vi "Main.vi"(11 "Module Admin":refnum<class "Delacor_lib_QMH_Module Admin.lvclass">) -> ()   [LabVIEW 2019, in "Controller.lvlib"]
doc: "This template is based off of the Queued Message Handler design pattern and the Queued Message Handler project template that ships with LabVIEW.\n\nThe main difference is that the queue is private to this module and communication between modules is performed via Broadcast and Request events.\n\nRequest events are wrapped in public API methods and are handled in the Event Handling Loop (EHL) of this VI. Any module can register for Broadcast events sent by this module. The EHL generates messages based on user interface actions.\n\nThe Message Handling Loop (MHL) processes messages generated by the EHL, or by other messages. The messages are string values, so new messages can be added easily to the Message Cases case structure in the MHL. Each message cluster can also provide an optional value for Message Data, which is a variant that can be converted to whatever message-specific data is required.\n_____\nBased on DQMH Project Template 6.0.0.91."
uses:
  Controller.lvlib
  <vilib>/Delacor/Delacor QMH/Libraries/Module Admin_class/Delacor_lib_QMH_Module Admin.lvclass
  Module Data--cluster.ctl
  <vilib>/Delacor/Delacor QMH/Libraries/Message Queue_class/Delacor_lib_QMH_Message Queue.lvclass/Delacor_lib_QMH_Message Queue.ctl
  Stop Argument--cluster.ctl
  <vilib>/Delacor/Delacor QMH/Libraries/Module Admin_class/Delacor_lib_QMH_Module Admin.lvclass/Delacor_lib_QMH_Module Admin.ctl
  <vilib>/Delacor/Delacor QMH/Libraries/Message Queue_class/Delacor_lib_QMH_Enqueue Message (Single).vi
  <vilib>/Delacor/Delacor QMH/Libraries/Module Admin_class/Delacor_lib_QMH_Get External Launch.vi
  <vilib>/Utility/error.llb/Error Cluster From Error Code.vi
  <vilib>/ErrorRing/Error Ring.xnode
  <vilib>/Delacor/Delacor QMH/Libraries/Message Queue_class/Delacor_lib_QMH_Message Queue.lvclass
  Server/Server.lvlib
panel:
  in  "Connect":bool
  in  "Disconnect":bool
  in  "Subpanel Ref":refnum<vi>
  out "Connected?":bool
  out "error out":errorcluster
  out "Status":string
  in  "Simulate MHL Error":bool
  in  "Simulate EHL Error":bool
  # "Controller"
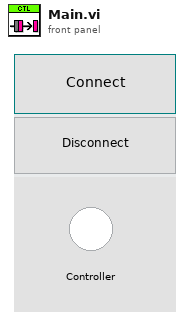
[diagram p1: front panel]
types:
  T1 = typedef "Controller.lvlib/Request Events--cluster.ctl" = cluster{"Stop Module":refnum<user-event>, "Show Panel":refnum<user-event>, "Hide Panel":refnum<user-event>, "Get Module Execution Status":refnum<user-event>, "Show Diagram":refnum<user-event>}
  T2 = typedef "Controller.lvlib/Module Data--cluster.ctl" = cluster{"Status":string}
  T3 = enum32{"invalid lock state", "Not Locked", "Locked (No Password)", "Password-protected"}
  T4 = typedef "Controller.lvlib/Stop Argument--cluster.ctl" = cluster{"Origin":string, "Exit via Stop Module Req?":bool, "Wait for Module to stop?":bool}
  T5 = enum32{"Invalid", "Standard", "Closed", "Hidden", "Minimized", "Maximized"}
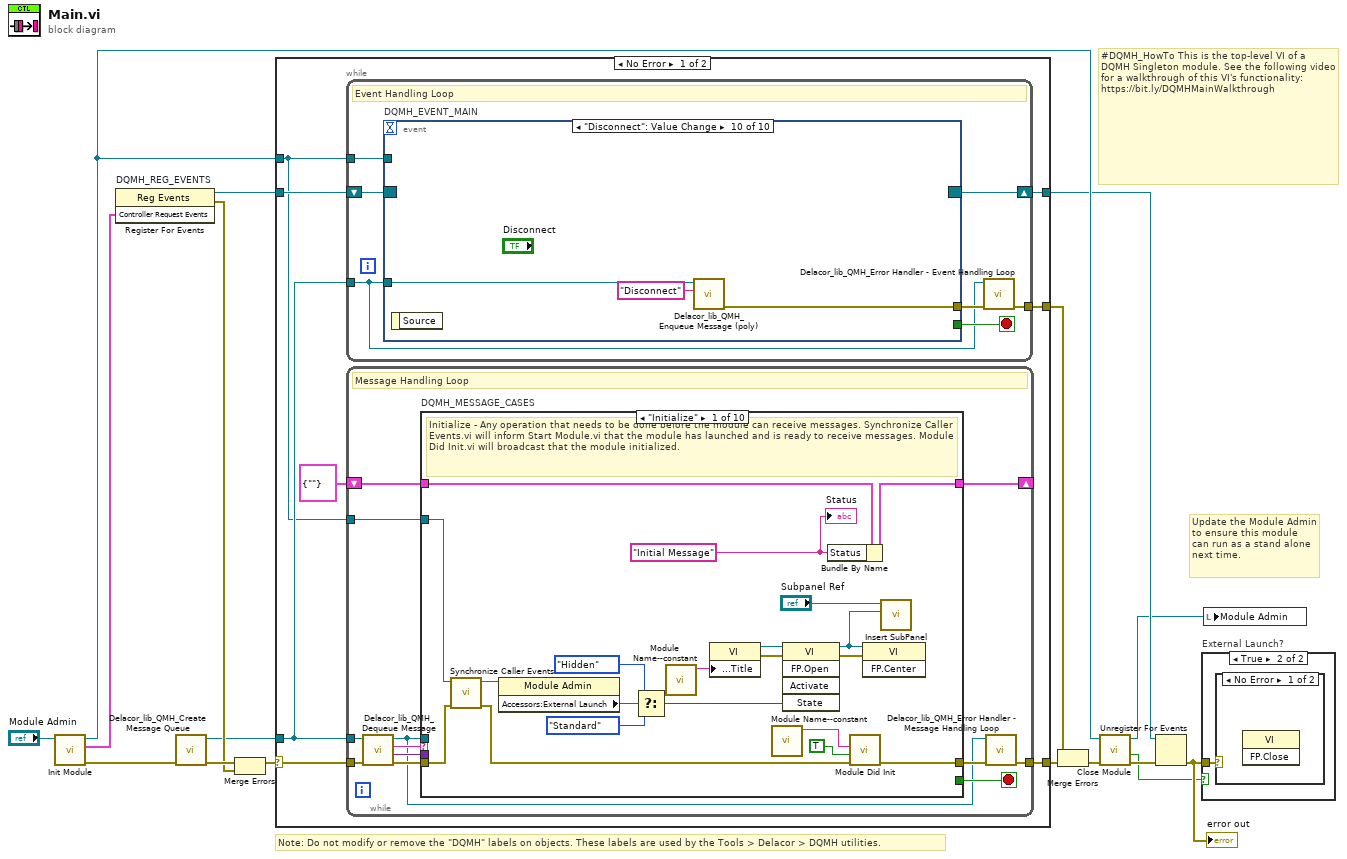
[diagram p0: block diagram]
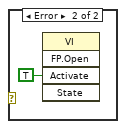
[diagram p3: hidden frame]
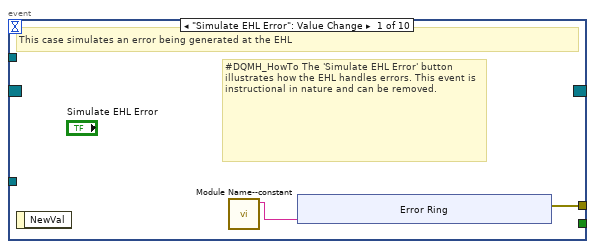
[diagram p4: hidden frame]
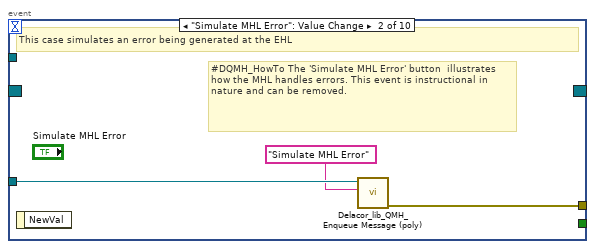
[diagram p5: hidden frame]
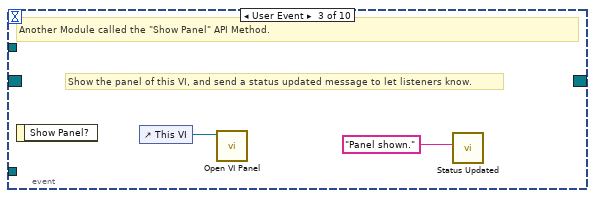
[diagram p6: hidden frame]
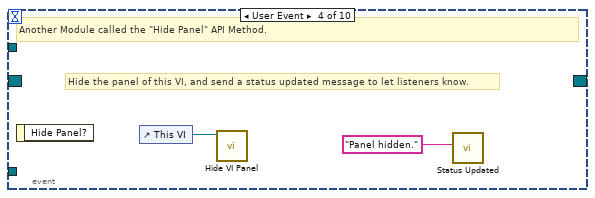
[diagram p7: hidden frame]
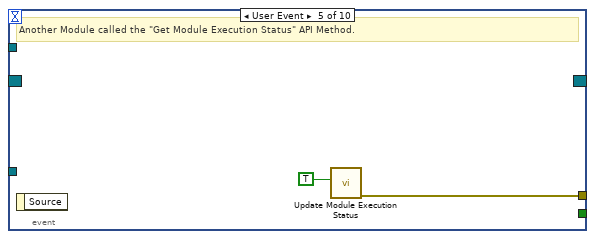
[diagram p8: hidden frame]
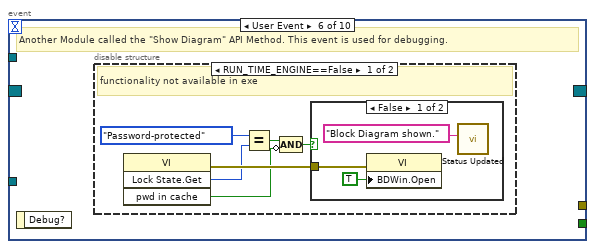
[diagram p9: hidden frame]
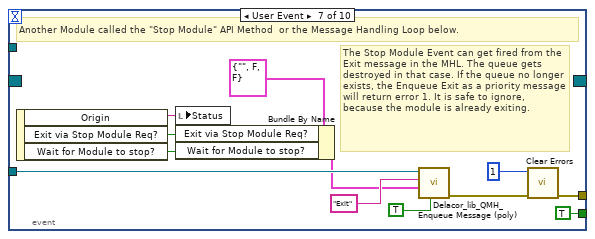
[diagram p12: hidden frame]
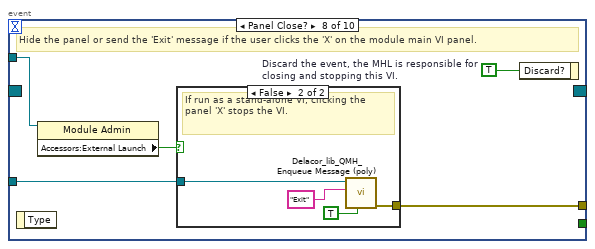
[diagram p13: hidden frame]
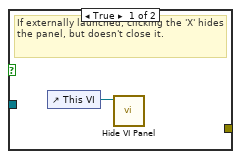
[diagram p14: hidden frame]
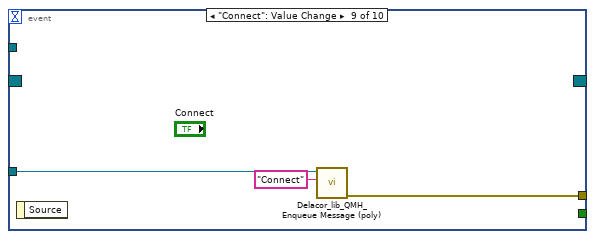
[diagram p15: hidden frame]
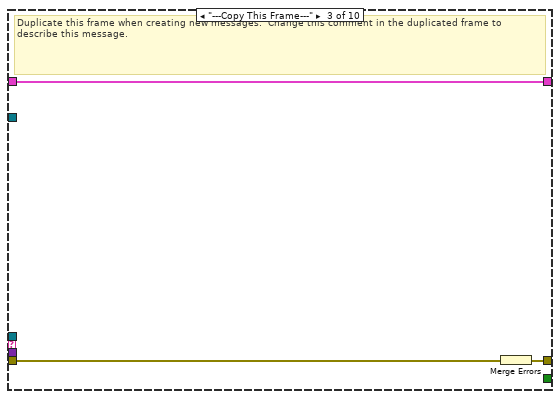
[diagram p17: hidden frame]
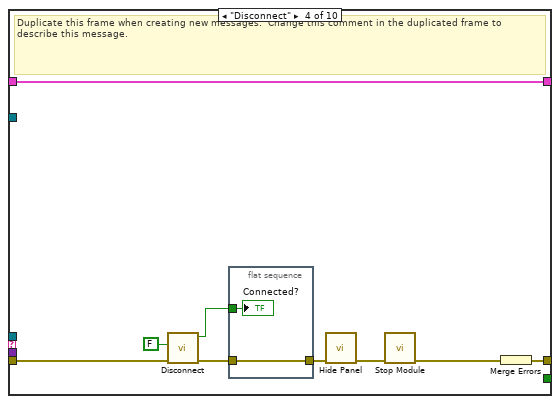
[diagram p18: hidden frame]
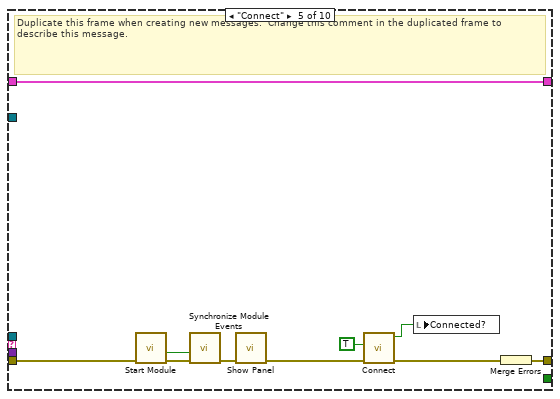
[diagram p19: hidden frame]
diagram:
  # "#DQMH_HowTo This is the top-level VI of a DQMH Singleton module. See the following video for a walkthrough of this VI's functionality: https://bit.ly/DQMHMainWalkthrough"
  # "Note: Do not modify or remove the \"DQMH\" labels on objects. These labels are used by the Tools > Delacor > DQMH utilities."
  # "Update the Module Admin to ensure this module can run as a stand alone next time."
  n1 = call "Init Module.vi"("Singleton Module Admin in"="Module Admin") -> ("error out"=w16:errorcluster, "Controller Request Events"=w5:T1, "Singleton Module Admin out"=w8:refnum<class "Delacor_lib_QMH_Module Admin.lvclass">)  [unwired: 8 in]
  n2 = register-events "DQMH_REG_EVENTS"(w5) -> (reference out=w6:refnum<event-registration>, error out=w9:errorcluster)  [unwired: 2 in]
  n3 = call <vilib>:"Delacor_lib_QMH_Create Message Queue.vi"("error in"=w16) -> ("error out"=w11:errorcluster, "Message Queue"=w4:refnum<class "Delacor_lib_QMH_Message Queue.lvclass">)  [unwired: 9 in]
  n4 = Merge Errors(w11, w9) -> (w10:errorcluster)
  n5 = case shown="No Error" w10 {
    selector: w10 -> [w23 w207]
    tunnel: [w25 w206] -> w17
    tunnel: [w22 w212] -> w7
    tunnel: w6 -> [w20 w212]
    tunnel: w4 -> [w19 w205]
    tunnel: [w24 _] -> w14
    tunnel: w8 -> [w18 w208]
    frame No Error {
      n6 = while {
        tunnel: w19 -> [w26]
        shift-right: [w29] -> w22
        shift-left: w20 -> [w30]
        tunnel: [w31] -> w24
        tunnel: w18 -> [w27]
        stop <- w28 stop-if-true
        # "Event Handling Loop"
        n7 = event "DQMH_EVENT_MAIN" shown="[9] \"Disconnect\": Value Change" {
          selector: w30 -> [_ _ _ _ _ _ _ _ _ _]
          dyn-events: [_ _ _ _ _ _ _ _ _ _] -> w29
          timeout: _ -> [_ _ _ _ _ _ _ _ _ _]
          tunnel: [_ _ _ _ _ _ TRUE ("Discard?") _ _ _] -> w28
          tunnel: w26 -> [_ w43 _ _ _ _ w67 w74 w84 w87]
          tunnel: [w34 w44 _ _ w50 _ w70 w76 w83 w86] -> w32
          tunnel: w27 -> [_ _ _ _ _ _ _ w73 _ _]
          event "Simulate EHL Error": Value Change {
            # "#DQMH_HowTo The 'Simulate EHL Error' button  illustrates how the EHL handles errors. This event is instructional in nature and can be removed."
            # "This case simulates an error being generated at the EHL"
            n8 = event-data() -> ()  [unwired: 1 in, 1 out]
            n9 = call "Module Name--constant.vi"() -> ("Module Name"=w33:string)  [unwired: 11 in]
            n10 = xnode "Error Ring"("parameter 0"=w33) -> ("error out"=w34:errorcluster)
          }
          event "Simulate MHL Error": Value Change {
            # "#DQMH_HowTo The 'Simulate MHL Error' button  illustrates how the MHL handles errors. This event is instructional in nature and can be removed."
            # "This case simulates an error being generated at the EHL"
            n11 = event-data() -> ()  [unwired: 1 in, 1 out]
            n12 = call-poly <vilib>:"Delacor_lib_QMH_Enqueue Message (poly).vi"("Message"="Simulate MHL Error", "Message Queue in"=w43) -> ("error out"=w44:errorcluster)  [unwired: 8 in, 1 out]
          }
          event User Event {
            # "Show the panel of this VI, and send a status updated message to let listeners know."
            # "Another Module called the \"Show Panel\" API Method."
            n13 = event-data() -> ()  [unwired: 1 in, 1 out]
            n14 = control-ref of="This VI"() -> (w46:refnum<vi>)
            n15 = call "Open VI Panel.vi"("VI"=w46) -> ()  [unwired: 10 in, 1 out]
            n16 = call "Status Updated.vi"("Status"="Panel shown." ("format string")) -> ()  [unwired: 10 in, 1 out]
          }
          event User Event {
            # "Hide the panel of this VI, and send a status updated message to let listeners know."
            # "Another Module called the \"Hide Panel\" API Method."
            n17 = event-data() -> ()  [unwired: 1 in, 1 out]
            n18 = control-ref of="This VI"() -> (w48:refnum<vi>)
            n19 = call "Hide VI Panel.vi"("VI"=w48) -> ()  [unwired: 10 in, 1 out]
            n20 = call "Status Updated.vi"("Status"="Panel hidden." ("format string")) -> ()  [unwired: 10 in, 1 out]
          }
          event User Event {
            # "Another Module called the \"Get Module Execution Status\" API Method."
            n21 = event-data() -> ()  [unwired: 1 in, 1 out]
            n22 = call "Update Module Execution Status.vi"("Running?"=TRUE) -> ("error out"=w50:errorcluster)  [unwired: 10 in]
          }
          event User Event {
            # "Another Module called the \"Show Diagram\" API Method. This event is used for debugging."
            n23 = event-data() -> ()  [unwired: 1 in, 1 out]
            n24 = disable-structure shown="RUN_TIME_ENGINE==False" {
              frame condition #0 (active) {
                # "functionality not available in exe"
                n25 = invoke class="VI" method="Lock State.Get"() -> (error out=w56:errorcluster, "Get Lock State"=w55:T3, "pwd in cache"=w52:bool)  [unwired: 4 in, 1 out]
                n26 = Equal?(x=T3."Password-protected", y=w55) -> (x = y?=w53:bool)
                n27 = Compound Arithmetic op=AND(w53, invert w52) -> (w51:bool)
                n28 = case shown="False" w51 {
                  tunnel: w56 -> [w59 _]
                  frame False {
                    n29 = property class="VI"(error in=w59, "BDWin.Open"=TRUE ("Block Diagram Window:Open")) -> ()  [unwired: 1 in, 2 out]
                    n30 = call "Status Updated.vi"("Status"="Block Diagram shown." ("format string")) -> ()  [unwired: 10 in, 1 out]
                  }
                  frame True {
                    # "Password-protected VI, and the password is not in the cache. Do not show the diagram."
                  }
                }
              }
              frame condition #1 {
              }
            }
          }
          event User Event {
            # "The Stop Module Event can get fired from the Exit message in the MHL. The queue gets destroyed in that case. If the queue no longer exists, the Enqueue Exit as a priority message will return error 1. It is safe to ignore, because the module is already exiting."
            # "Another Module called the \"Stop Module\" API Method  or the Message Handling Loop below."
            n31 = event-data() -> ("Origin"=w66:string, "Exit via Stop Module Req?"=w62:bool, "Wait for Module to stop?"=w61:bool)  [unwired: 1 in]
            n32 = local write "Status"(w66) -> ()
            n33 = Bundle By Name(cluster=T4 {"Origin"="", "Exit via Stop Module Req?"=FALSE, "Wait for Module to stop?"=FALSE} ("Stop Argument"), "Exit via Stop Module Req?"=w62, "Wait for Module to stop?"=w61) -> (w60:T4)
            n34 = call-poly <vilib>:"Delacor_lib_QMH_Enqueue Message (poly).vi"("Priority Message? (F)"=TRUE, "Message Data"=w60, "Message"="Exit", "Message Queue in"=w67) -> ("error out"=w71:errorcluster)  [unwired: 6 in, 1 out]
            n35 = call <vilib>:"Clear Errors.vi"("error in (no error)"=w71, "specific error code to clear (0: all)"=1) -> ("error out"=w70:errorcluster)  [unwired: 4 in, 1 out]
          }
          event Panel Close? {
            w75 = TRUE  # Discard the event, the MHL is responsible for closing and stopping this VI.
            # "Hide the panel or send the 'Exit' message if the user clicks the 'X' on the module main VI panel."
            n36 = event-data() -> ()  [unwired: 1 in, 1 out]
            n37 = property class="Module Admin"(reference=w73) -> ("Accessors:External Launch"=w72:bool)  [unwired: 1 in, 2 out]
            n38 = case shown="False" w72 {
              tunnel: w74 -> [_ w80]
              tunnel: [_ w81] -> w76
              frame True {
                # "If externally launched, clicking the 'X' hides the panel, but doesn't close it."
                n39 = control-ref of="This VI"() -> (w77:refnum<vi>)
                n40 = call "Hide VI Panel.vi"("VI"=w77) -> ()  [unwired: 10 in, 1 out]
              }
              frame False {
                # "If run as a stand-alone VI, clicking the panel 'X' stops the VI."
                n41 = call-poly <vilib>:"Delacor_lib_QMH_Enqueue Message (poly).vi"("Priority Message? (F)"=TRUE, "Message"="Exit", "Message Queue in"=w80) -> ("error out"=w81:errorcluster)  [unwired: 7 in, 1 out]
              }
            }
            n42 = event-data("Discard?"=w75) -> ()  [unwired: 1 in, 1 out]
          }
          event "Connect": Value Change {
            n43 = event-data() -> ()  [unwired: 1 in, 1 out]
            n44 = call-poly <vilib>:"Delacor_lib_QMH_Enqueue Message (poly).vi"("Message"="Connect", "Message Queue in"=w84) -> ("error out"=w83:errorcluster)  [unwired: 8 in, 1 out]
          }
          event "Disconnect": Value Change {
            n45 = event-data() -> ()  [unwired: 1 in, 1 out]
            n46 = call-poly <vilib>:"Delacor_lib_QMH_Enqueue Message (poly).vi"("Message"="Disconnect", "Message Queue in"=w87) -> ("error out"=w86:errorcluster)  [unwired: 8 in, 1 out]
          }
        }
        n47 = call-dynamic "Delacor_lib_QMH_Error Handler - Event Handling Loop.vi"("error in"=w32, "Message Queue in"=w26) -> ("dup error in"=w31:errorcluster)  [unwired: 8 in, 1 out]
      }
      n48 = while {
        tunnel: w19 -> [w90]
        shift-right: [w94] -> _
        shift-left: T2 {"Status"=""} ("Data Cluster") -> [w95]
        tunnel: w23 -> [w98]
        tunnel: [w96] -> w25
        tunnel: w18 -> [w88]
        stop <- w93 stop-if-true
        # "Message Handling Loop"
        n49 = call-dynamic "Delacor_lib_QMH_Dequeue Message.vi"("error in"=w98, "Message Queue in"=w90) -> ("error out"=w97:errorcluster, "Message Data"=w91:variant, "Message"=w92:string, "Message Queue out"=w89:refnum<class "Delacor_lib_QMH_Message Queue.lvclass">)  [unwired: 6 in]
        n50 = case "DQMH_MESSAGE_CASES" shown="\"Initialize\"" w92 {
          selector: w92 -> [_ _ _ _ _ _ _ _ _ w192]
          tunnel: w89 -> [_ _ _ _ _ _ _ w162 w184 _]
          tunnel: w97 -> [w117 w121 w124 w131 w139 w147 w152 w169 w190 w194]
          tunnel: [w115 w121 w123 w133 w145 w147 w151 w165 w187 w195] -> w99
          tunnel: w95 -> [w107 w120 w122 w132 w144 w146 w149 w164 w183 w193]
          tunnel: [w106 w120 w122 w132 w144 w146 w149 w164 w183 w193] -> w94
          tunnel: [_ _ _ _ _ _ _ _ w182 _] -> w93
          tunnel: w91 -> [_ _ _ _ _ _ _ w163 w181 _]
          tunnel: w88 -> [w108 _ _ _ _ _ _ w161 w176 _]
          frame "Initialize" {
            w102 = "Initial Message" ("Initial Message")
            # "Initialize - Any operation that needs to be done before the module can receive messages. Synchronize Caller Events.vi will inform Start Module.vi that the module has launched and is ready to receive messages. Module Did Init.vi will broadcast that the module initialized."
            n51 = call "Synchronize Caller Events.vi"("error in (no error)"=w117, "Singleton Module Admin in"=w108) -> ("error out"=w116:errorcluster, "Singleton Module Admin out"=w103:refnum<class "Delacor_lib_QMH_Module Admin.lvclass">)  [unwired: 8 in]
            n52 = property class="Module Admin"(reference=w103) -> ("Accessors:External Launch"=w112:bool)  [unwired: 1 in, 2 out]
            n53 = Select(t=T5."Hidden" ("State"), s=w112, f=T5."Standard" ("State")) -> (s? t:f=w109:T5)
            n54 = call "Module Name--constant.vi"() -> ("Module Name"=w114:string)  [unwired: 11 in]
            n55 = property class="VI"("Front Panel.Title"=w114) -> (reference out=w113:refnum<vi>, error out=w119:errorcluster)  [unwired: 2 in]
            n56 = call "Module Name--constant.vi"() -> ("Module Name"=w104:string)  [unwired: 11 in]
            n57 = invoke class="VI" method="FP.Open"(reference=w113, error in=w119, "State"=w109) -> (reference out=w101:refnum<vi>, error out=w118:errorcluster)  [unwired: 2 in, 3 out]
            n58 = Bundle By Name(cluster=w107, "Status"=w102) -> (w106:T2)
            n59 = call "Module Did Init.vi"("error in (no error)"=w116, "Initialized?"=TRUE, "Origin"=w104) -> ("error out"=w115:errorcluster)  [unwired: 8 in]
            n60 = invoke class="VI" method="FP.Center"(reference=w101, error in=w118) -> ()  [unwired: 1 in, 3 out]
            n61 = call "Insert SubPanel.vi"("VI Ref"=w101, "Subpanel Ref"="Subpanel Ref") -> ()  [unwired: 9 in, 1 out]
            "Status" <- w102
          }
          frame "---Module Specific---" {
            # "Separator -- The following cases handle messages specific to this Module."
          }
          frame "---Copy This Frame---" {
            # "Duplicate this frame when creating new messages.  Change this comment in the duplicated frame to describe this message."
            n62 = Merge Errors(w124) -> (w123:errorcluster)
          }
          frame "Disconnect" {
            # "Duplicate this frame when creating new messages.  Change this comment in the duplicated frame to describe this message."
            n63 = call "Disconnect.vi"("error in"=w131, "Disconnect"=FALSE) -> ("error out"=w126:errorcluster, "Connected?"=w129:bool)  [unwired: 7 in, 1 out]
            n64 = flat-sequence {
              tunnel: w129 -> [w135]
              tunnel: w126 -> [w134]
              tunnel: [w134] -> w125
              frame #0 {
                "Connected?" <- w135
              }
            }
            n65 = call "Hide Panel.vi"("error in (no error)"=w125) -> ("error out"=w128:errorcluster)  [unwired: 10 in]
            n66 = call "Stop Module.vi"("error in"=w128) -> ("error out"=w127:errorcluster)  [unwired: 10 in]
            n67 = Merge Errors(w127) -> (w133:errorcluster)
          }
          frame "Connect" {
            # "Duplicate this frame when creating new messages.  Change this comment in the duplicated frame to describe this message."
            n68 = call "Start Module.vi"("error in (no error)"=w139) -> ("error out"=w140:errorcluster, "Wait for Event Sync?"=w138:bool)  [unwired: 7 in, 2 out]
            n69 = call "Synchronize Module Events.vi"("error in"=w140, "Wait for Event Sync?"=w138) -> ("error out"=w137:errorcluster)  [unwired: 9 in]
            n70 = call "Show Panel.vi"("error in (no error)"=w137) -> ("error out"=w136:errorcluster)  [unwired: 10 in]
            n71 = call "Connect.vi"("error in"=w136, "Connect"=TRUE) -> ("error out"=w142:errorcluster, "Connected?"=w141:bool)  [unwired: 7 in, 1 out]
            n72 = local write "Connected?"(w141) -> ()
            n73 = Merge Errors(w142) -> (w145:errorcluster)
          }
          frame "---Exit and Error Handling---" {
            # "Separator - The following cases handle errors and exit messages."
          }
          frame "Simulate MHL Error" {
            # "#DQMH_HowTo The 'Simulate MHL Error' button  illustrates how the MHL handles errors. This event is instructional in nature and can be removed."
            # "Simulate an error occurring at the MHL"
            n74 = call "Module Name--constant.vi"() -> ("Module Name"=w148:string)  [unwired: 11 in]
            n75 = xnode "Error Ring"("parameter 0"=w148) -> ("error out"=w150:errorcluster)
            n76 = Merge Errors(w152, w150) -> (w151:errorcluster)
          }
          frame "Error" {
            # "#CodeRecommended - If you ever change the name of this \"Error\" message, you'll need to update the name in the Check Loop Error.vi as well."
            # "#CodeRecommended - If the module is running in standalone mode (External Launch = FALSE), this code will pop up an error dialog and call the 'Exit' message if an error occurs. Add more fine-grained error handling here."
            # "Error - Check the error message data and respond accordingly. This message is sent by the \"Error Handler\" VIs at the end of each loop in this application."
            n77 = property class="Module Admin"(reference=w161) -> ("Accessors:External Launch"=w160:bool)  [unwired: 1 in, 2 out]
            n78 = Variant To Data(error in=w169, type=errorcluster {"status"=FALSE, "code"=0, "source"=""} ("error constant"), Variant=w163) -> (data=w170:errorcluster, error out=w167:errorcluster)
            n79 = call "Error Reported.vi"("Error"=w170) -> ()  [unwired: 10 in, 1 out]
            n80 = case shown="False" w160 {
              tunnel: [w175 _] -> w166
              tunnel: w162 -> [w173 _]
              tunnel: w170 -> [w174 _]
              frame False {
                # "If the module is running standalone, then pop up an error dialog and call the \"Exit\" message."
                n81 = call <vilib>:"Simple Error Handler.vi"("error in (no error)"=w174) -> ()  [unwired: 4 in, 5 out]
                n82 = call-poly <vilib>:"Delacor_lib_QMH_Enqueue Message (poly).vi"("Priority Message? (F)"=TRUE, "Message"="Exit", "Message Queue in"=w173) -> ("error out"=w175:errorcluster)  [unwired: 7 in, 1 out]
              }
              frame True {
                # "If the module was launched externally, calling the Error Reported broadcast VI is the only action performed by the \"Error\" message. The module's caller can then process the error appropriately."
              }
            }
            n83 = Merge Errors(w167, w166) -> (w165:errorcluster)
            n84 = local write "error out"(w165) -> ()
          }
          frame "Exit" {
            w180 = 91  # 91: not all Exit messages will have an argument
            w182 = TRUE  # Stop the VI
            # "Release the message queue reference"
            # "#CodeNeeded - Add any required cleanup code here"
            # "Exit - Exit the application."
            n85 = Variant To Data(error in=w190, type=T4 {"Origin"="", "Exit via Stop Module Req?"=FALSE, "Wait for Module to stop?"=FALSE} ("Stop Argument"), Variant=w181) -> (data=w178:T4, error out=w186:errorcluster)
            n86 = call <vilib>:"Clear Errors.vi"("error in (no error)"=w186, "specific error code to clear (0: all)"=w180) -> ("error out"=w189:errorcluster)  [unwired: 4 in, 1 out]
            n87 = control-ref of="This VI"() -> (w177:refnum<vi>)
            n88 = call-dynamic "Delacor_lib_QMH_Release Message Queue.vi"("error in"=w189, "Message Queue"=w184) -> ("error out"=w188:errorcluster)  [unwired: 9 in]
            n89 = call "Handle Exit.vi"("Stop Argument"=w178, "Admin in"=w176, "VI reference"=w177) -> ("error out"=w185:errorcluster)  [unwired: 7 in, 1 out]
            n90 = Merge Errors(w188, w185) -> (w187:errorcluster)
          }
          frame Default {
            # "'Default' case only runs if there is a message that isn't defined in any of the other cases.  Output a programming error."
            n91 = call "Module Name--constant.vi"() -> ("Module Name"=w191:string)  [unwired: 11 in]
            n92 = xnode "Error Ring"("parameter 0"=w192, "parameter 1"=w191) -> ("error out"=w196:errorcluster)
            n93 = Merge Errors(w194, w196) -> (w195:errorcluster)
          }
        }
        n94 = call-dynamic "Delacor_lib_QMH_Error Handler - Message Handling Loop.vi"("error in"=w99, "Message Queue in"=w89) -> ("dup error in"=w96:errorcluster)  [unwired: 8 in, 1 out]
      }
    }
    frame Error {
      # "Synchronize Caller Events.vi will inform Start Module.vi that the module has launched and will let the code calling Start Module.vi register for broadcasts and would permit the caller receive the broadcast that an error occurred at launch time."
      n95 = call-dynamic "Delacor_lib_QMH_Release Message Queue.vi"("error in"=w207, "Message Queue"=w205) -> ("error out"=w206:errorcluster)  [unwired: 9 in]
      n96 = call "Synchronize Caller Events.vi"("Singleton Module Admin in"=w208) -> ("error out"=w213:errorcluster)  [unwired: 9 in, 1 out]
      n97 = call "Module Name--constant.vi"() -> ("Module Name"=w211:string)  [unwired: 11 in]
      n98 = Format Into String(format string="An error occurred during initialization. %s is no longer running.", w211) -> (resulting string=w209:string)  [unwired: 2 in, 1 out]
      n99 = Merge Errors(w206, w213) -> (w214:errorcluster)
      n100 = call "Error Reported.vi"("Additional Information"=w209, "Error"=w214) -> ()  [unwired: 9 in, 1 out]
    }
  }
  n101 = Merge Errors(w14, w17) -> (w13:errorcluster)
  n102 = call "Close Module.vi"("error in (no error)"=w13, "Module Admin in"=w8) -> ("error out"=w15:errorcluster, "External Launch"=w1:bool, "Module Admin out"=w2:refnum<class "Delacor_lib_QMH_Module Admin.lvclass">)  [unwired: 7 in]
  n103 = Unregister For Events(event registration refnum=w7, error in=w15) -> (error out=w12:errorcluster)
  "error out" <- w12
  n104 = case "External Launch?" shown="True" w1 {
    tunnel: w12 -> [_ w215]
    frame False {
    }
    frame True {
      n105 = case shown="No Error" w215 {
        frame No Error {
          n106 = invoke class="VI" method="FP.Close"() -> ()  [unwired: 3 in, 3 out]
        }
        frame Error {
          n107 = invoke class="VI" method="FP.Open"("Activate"=TRUE ("Activate?")) -> ()  [unwired: 4 in, 5 out]
        }
      }
    }
  }
  n108 = local write "Module Admin"(w2) -> ()
